vi "Initialise Standard Display.vi"() -> (3 "Standard Display Configuration out":refnum<class "Standard Display Configuration.lvclass">)   [LabVIEW 2016, in "Assert API Components.lvlib" / "Assert Display.lvlib" / "Main Display.lvlib" / "Standard Display Configuration.lvclass"]
doc: "Creates a new instance of the standard display configuration class with a variant for storing the list of assert names in."
uses:
  Standard Display Configuration.lvclass
  C:/Users/ukhornp/Documents/Projects/actor_assert_api/Core/Main Display/Display Configurations/Base Display Configuration.lvclass
  Base Display Configuration.lvclass/Base Display Configuration.ctl
  Base Display Configuration.lvclass
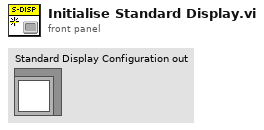
[diagram p1: front panel]
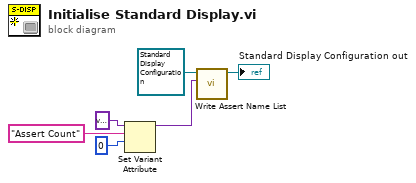
[diagram p0: block diagram]
diagram:
  n1 = Set Variant Attribute(Variant=variant ("Assert Name List"), name="Assert Count", value=0) -> (Variant out=w4:variant)  [unwired: 1 in, 2 out]
  n2 = call "Write Assert Name List.vi"("Assert Name List"=w4, "Base Display Configuration in"=refnum<class "Standard Display Configuration.lvclass"> refnum ("Standard Display Configuration in")) -> ("Base Display Configuration out"=→"Standard Display Configuration out":refnum<class "Standard Display Configuration.lvclass">)  [unwired: 9 in]
